vi "umSnapToHz.vi"(8 "error in (no error)":errorcluster, 11 "Snap Buffer (um) in":u64[](array[numeric])) -> (0 "error out":errorcluster, 2 "Frame Rate (Hz)":dbl, 3 "Snap Buffer(um) out":u64[](array[numeric]))   [LabVIEW 2020]
uses:
  _controls/Timer_actions.ctl
  <vilib>/Analysis/baseanly.llb/Mean (DBL).vi
  <vilib>/Analysis/NI_AALBase.lvlib
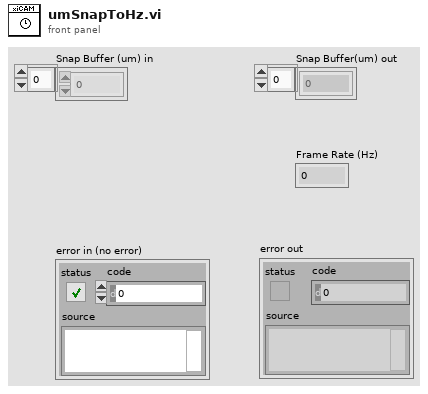
[diagram p1: front panel]
types:
  T1 = typedef "Timer_actions.ctl" = enum16{"Reset", "Snap", "Total"}
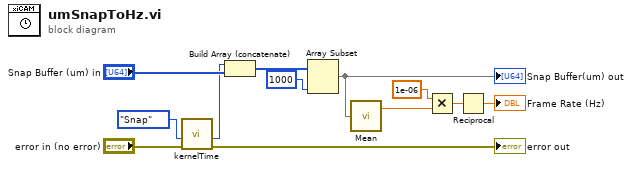
[diagram p0: block diagram]
diagram:
  n1 = call "kernelTime.vi"("error in (no error) in"="error in (no error)", "Action (Snap)"=Timer_actions."Snap") -> ("error out"=→"error out":errorcluster, "Microseconds"=w2:u64)  [unwired: 8 in]
  n2 = Build Array (concatenate)(w2, "Snap Buffer (um) in") -> (w7:u64[])
  n3 = Array Subset(array=w7, length=1000) -> (w9:u64[])  [unwired: 1 in]
  "Snap Buffer(um) out" <- w9
  n4 = call-poly <vilib>:"Mean.vi"("X"=w9) -> ("mean"=w6:dbl)  [unwired: 1 out]
  n5 = Multiply(x=1e-06, y=w6) -> (x*y=w10:dbl)
  n6 = Reciprocal(x=w10) -> (1/x=→"Frame Rate (Hz)":dbl)
